vi "Approximately equals.vi"   [LabVIEW 2011, in "COSYLib.lvlib"]
doc: "Returns TRUE if x falls within the range (y-dy, y+dy)."
uses:
  COSYLib.lvlib
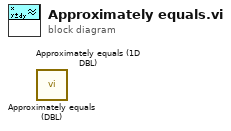
[diagram p0: block diagram]
diagram:
  n1 = call "Approximately equals (DBL).vi"() -> ()  [unwired: 11 in, 1 out]
  n2 = call "Approximately equals (1D DBL).vi"() -> ()  [unwired: 11 in, 1 out]
